vi "Stop DAQ Tasks.vi"(8 "error in (no error)":errorcluster, 11 "LockinDAQ in":refnum<class "LockinDAQ.lvclass">) -> (0 "error out":errorcluster, 3 "LockinDAQ out":refnum<class "LockinDAQ.lvclass">)   [LabVIEW 2016, in "LockinDAQ.lvclass"]
uses:
  LockinDAQ.lvclass
  LockinDAQ.lvclass/LockinDAQ.ctl
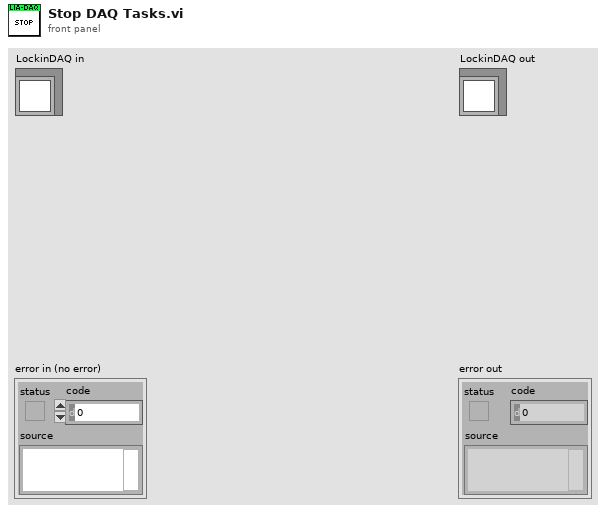
[diagram p1: front panel]
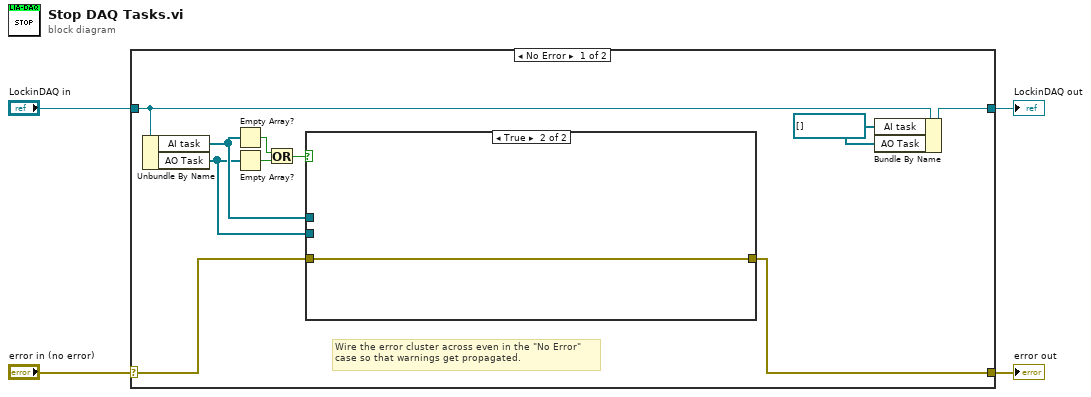
[diagram p0: block diagram]
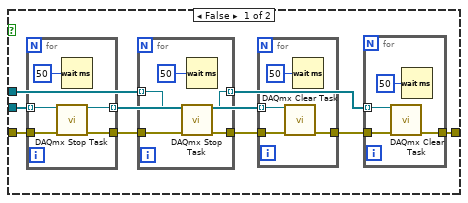
[diagram p2: hidden frame]
diagram:
  n1 = case shown="No Error" "error in (no error)" {
    selector: "error in (no error)" -> [w14 w44]
    tunnel: [w8 w44] -> w3
    tunnel: [w7 w43] -> w1
    tunnel: "LockinDAQ in" -> [w5 w43]
    frame No Error {
      w6 = refnum<k21>[] [] ("AI task")
      # "Wire the error cluster across even in the \"No Error\"\ncase so that warnings get propagated."
      n2 = Unbundle By Name(w5) -> ("AI task"=w13:refnum<k21>[], "AO Task"=w12:refnum<k21>[])
      n3 = Empty Array?(array=w13) -> (empty?=w10:bool)
      n4 = Empty Array?(array=w12) -> (empty?=w11:bool)
      n5 = Or(x=w10, y=w11) -> (x .or. y?=w9:bool)
      n6 = case shown="True" w9 {
        tunnel: w14 -> [w18 w42]
        tunnel: w13 -> [w16 _]
        tunnel: w12 -> [w15 _]
        tunnel: [w17 w42] -> w8
        frame False {
          n7 = for {
            tunnel: w15 -> [w41] mode=indexing
            tunnel: [w39] -> w19 mode=indexing
            tunnel: w18 -> [w38]
            tunnel: [w37] -> w22
            n8 = call <vilib>:"DAQmx Stop Task.vi"("task/channels in"=w41, "error in"=w38) -> ("task out"=w39:refnum<k21>, "error out"=w37:errorcluster)  [unwired: 12 in]
            n9 = Wait (ms)(milliseconds to wait=u32 50) -> ()  [unwired: 1 out]
          }
          n10 = for {
            tunnel: w16 -> [w36] mode=indexing
            tunnel: [w34] -> w23 mode=indexing
            tunnel: w22 -> [w33]
            tunnel: [w32] -> w20
            n11 = call <vilib>:"DAQmx Stop Task.vi"("task/channels in"=w36, "error in"=w33) -> ("task out"=w34:refnum<k21>, "error out"=w32:errorcluster)  [unwired: 12 in]
            n12 = Wait (ms)(milliseconds to wait=u32 50) -> ()  [unwired: 1 out]
          }
          n13 = for {
            tunnel: w19 -> [w31] mode=indexing
            tunnel: w20 -> [w29]
            tunnel: [w28] -> w21
            n14 = call <vilib>:"DAQmx Clear Task.vi"("task in"=w31, "error in"=w29) -> ("error out"=w28:errorcluster)  [unwired: 13 in]
            n15 = Wait (ms)(milliseconds to wait=u32 50) -> ()  [unwired: 1 out]
          }
          n16 = for {
            tunnel: w23 -> [w27] mode=indexing
            tunnel: w21 -> [w25]
            tunnel: [w24] -> w17
            n17 = call <vilib>:"DAQmx Clear Task.vi"("task in"=w27, "error in"=w25) -> ("error out"=w24:errorcluster)  [unwired: 13 in]
            n18 = Wait (ms)(milliseconds to wait=u32 50) -> ()  [unwired: 1 out]
          }
        }
        frame True {
        }
      }
      n19 = Bundle By Name(cluster=w5, "AI task"=w6, "AO Task"=w6) -> (w7:refnum<class "LockinDAQ.lvclass">)
    }
    frame Error {
    }
  }
  "error out" <- w3
  "LockinDAQ out" <- w1
